vi "removeServer.vi"(8 "error in (no error)":errorcluster, 10 "Remove Server in":refnum<class "IServer.lvclass">, 11 "IDevice in":refnum<class "IDevice.lvclass">) -> (0 "error out":errorcluster, 2 "Remove Server out":refnum<class "IServer.lvclass">, 3 "IDevice out":refnum<class "IDevice.lvclass">)   [LabVIEW 2022 SP3, in "openDAQ.lvlib" / "IBaseObject.lvlib" / "IPropertyObject.lvlib" / "IComponent.lvlib" / "IFolder.lvlib" / "IDevice.lvlib" / "IDevice.lvclass"]
uses:
  <instrlib>/openDAQ/Public/Classes/IDevice/IDevice.lvclass
  <instrlib>/openDAQ/Public/Classes/IDevice/IDevice.lvclass/IDevice.ctl
  <instrlib>/openDAQ/Public/Classes/IServer/IServer.lvclass
  <instrlib>/openDAQ/Binaries/Windows/x86/copendaq32.dll
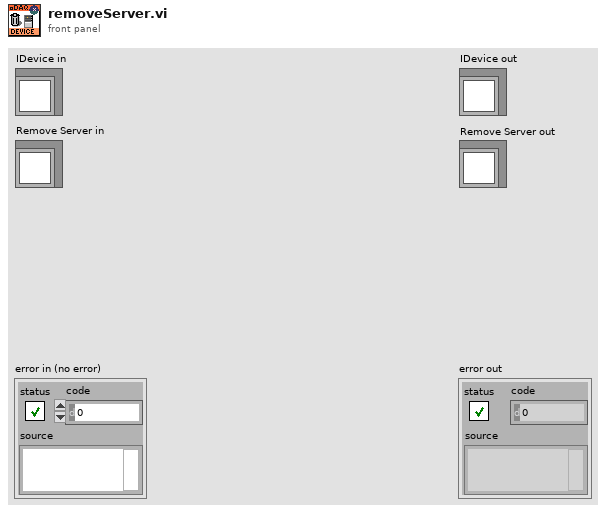
[diagram p1: front panel]
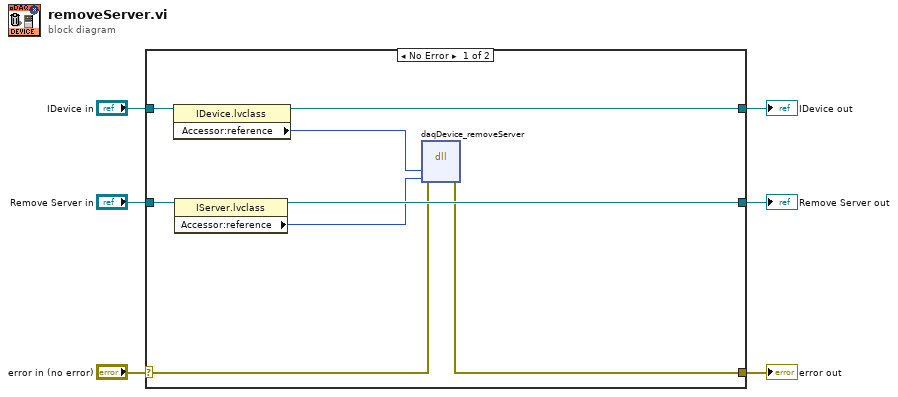
[diagram p0: block diagram]
diagram:
  n1 = case shown="No Error" "error in (no error)" {
    selector: "error in (no error)" -> [w11 w17]
    tunnel: [w10 w17] -> w5
    tunnel: [w9 w16] -> w3
    tunnel: "IDevice in" -> [w13 w16]
    tunnel: "Remove Server in" -> [w8 w15]
    tunnel: [w14 w15] -> w1
    frame No Error {
      n2 = property class="IDevice.lvclass"(reference=w13) -> (reference out=w9:refnum<class "IDevice.lvclass">, "Accessor:reference"=w12:i64)  [unwired: 1 in, 1 out]
      n3 = property class="IServer.lvclass"(reference=w8) -> (reference out=w14:refnum<class "IServer.lvclass">, "Accessor:reference"=w7:i64)  [unwired: 1 in, 1 out]
      n4 = dll-call lib="C:/Program Files (x86)/National Instruments/LabVIEW 2022/instr.lib/openDAQ/Binaries/Windows/x86/copendaq*.*" fn="daqDevice_removeServer"(error in=w11, "device"=w12, "removeServer"=w7) -> (error out=w10:errorcluster)  [unwired: 5 in, 1 out]
    }
    frame Error {
    }
  }
  "error out" <- w5
  "IDevice out" <- w3
  "Remove Server out" <- w1
